vi "data type tester.vi"() -> ()   [LabVIEW 2015]
panel:
  out "double precision float":dbl
  in  "Numeric":i16
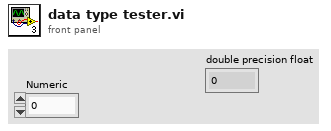
[diagram p1: front panel]
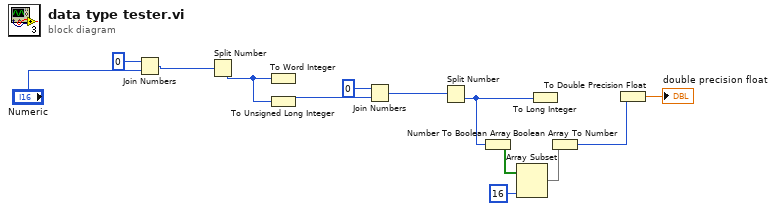
[diagram p0: block diagram]
diagram:
  n1 = Join Numbers(hi=i16 0, lo="Numeric") -> ((hi.lo)=w11:u32)
  n2 = Split Number(x=w11) -> (lo(x)=w10:u16)  [unwired: 1 out]
  n3 = To Word Integer(number=w10) -> ()  [unwired: 1 out]
  n4 = To Unsigned Long Integer(number=w10) -> (unsigned 32bit integer=w9:u32)
  n5 = Join Numbers(hi=u32 0, lo=w9) -> ((hi.lo)=w7:u64)
  n6 = Split Number(x=w7) -> (lo(x)=w5:u32)  [unwired: 1 out]
  n7 = Number To Boolean Array(number=w5) -> (Boolean array=w3:bool[])
  n8 = Array Subset(array=w3, length=16) -> (w1:bool[])  [unwired: 1 in]
  n9 = To Long Integer(number=w5) -> ()  [unwired: 1 out]
  n10 = Boolean Array To Number(Boolean array=w1) -> (number=w4:i32)
  n11 = To Double Precision Float(number=w4) -> (double precision float=→"double precision float":dbl)
